vi "ServoLatch.vi"(10 "Button X Hit":bool) -> ()   [LabVIEW 2012]
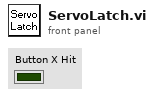
[diagram p1: front panel]
types:
  T1 = typedef "WPI_ServoDeviceRef.ctl" = cluster{"DeviceStatus":errorcluster, "Digital Module":T2, "PWM Channel":T3, "DeadBand":T4}
  T2 = typedef "FPGA_TypedefDigitalModule.ctl" = enum16{"Digital Module 1", "Digital Module 2"}
  T3 = typedef "FPGA_DIOPWMChannel.ctl" = enum8{"PWM 1", "PWM 2", "PWM 3", "PWM 4", "PWM 5", "PWM 6", "PWM 7", "PWM 8", "PWM 9", "PWM 10", "Invalid"}
  T4 = typedef "WPI_PWMDeadband.ctl" = cluster{"Name":string, "maxPositivePwm":i32, "minPositivePwm":i32, "centerPwm":i32, "maxNegativePwm":i32, "minNegativePwm":i32, "angularRange":u16}
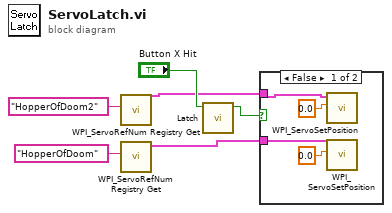
[diagram p0: block diagram]
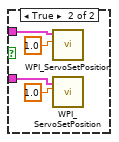
[diagram p2: hidden frame]
diagram:
  n1 = call <vilib>:"WPI_ServoRefNum Registry Get.vi"("refnum name"="HopperOfDoom2") -> ("ServoDeviceRef"=w2:T1)  [unwired: 9 in, 1 out]
  n2 = call <vilib>:"WPI_ServoRefNum Registry Get.vi"("refnum name"="HopperOfDoom") -> ("ServoDeviceRef"=w1:T1)  [unwired: 9 in, 1 out]
  n3 = call "Latch.vi"("Latch In"="Button X Hit") -> ("Latch Out"=w4:bool)  [unwired: 10 in]
  n4 = case shown="False" w4 {
    tunnel: w2 -> [w8 w12]
    tunnel: w1 -> [w7 w11]
    frame False {
      n5 = call <vilib>:"WPI_ServoSetPosition.vi"("Position"=0.0, "ServoDeviceRef"=w8) -> ()  [unwired: 8 in, 2 out]
      n6 = call <vilib>:"WPI_ServoSetPosition.vi"("Position"=0.0, "ServoDeviceRef"=w7) -> ()  [unwired: 8 in, 2 out]
    }
    frame True {
      n7 = call <vilib>:"WPI_ServoSetPosition.vi"("Position"=1.0, "ServoDeviceRef"=w12) -> ()  [unwired: 8 in, 2 out]
      n8 = call <vilib>:"WPI_ServoSetPosition.vi"("Position"=1.0, "ServoDeviceRef"=w11) -> ()  [unwired: 8 in, 2 out]
    }
  }
